vi "Kinematics_Wheel Deltas to Twist.vi"(9 "WheelDeltas":T2[](array[typedef]) {"Angle"."SIN" format="%13.4f"; "Angle"."COS" format="%13.4f"; "Angle"."VALUE" format="%13.4f"}, 11 "In SWERVE_DRIVE_KINEMATICS":T4 {"SavedModuleStates"."Angle"."SIN" format="%13.4f"; "SavedModuleStates"."Angle"."COS" format="%13.4f"; "SavedModuleStates"."Angle"."VALUE" format="%13.4f"; "PrevCoR"."Y" format="%14.3f"; "PrevCoR"."X" format="%14.3f"; "Modules"."Y" format="%14.3f"; "Modules"."X" format="%14.3f"}) -> (1 "Size Error Out":bool, 3 "Twist2d Out":T1)   [LabVIEW 2023, in "Swerve_Odometry_SEN.lvlib"]
doc: "Performs forward kinematics to return the resulting chassis state from the given module states. This method is often used for odometry -- determining the robot's position on the field using data from the real-world speed and angle of each module on the robot.\n\n\nParameters: \n - in Swerve Drive Kinematics - Swerve drive kinematics data structure\n - wheelDeltas - An array of the latest change in position of the modules (as a SwerveModulePosition type) as measured from respective encoders and gyros. The order of the swerve module states should be same as passed into the constructor of this class.\n\nReturns:\n - The resulting twist2d."
uses:
  Swerve_Odometry_SEN.lvlib
  Cluster_SWERVE_DRIVE_KINEMATICS.ctl
  <vilib>/Analysis/Matrix/Datatypes/RealMatrix.ctl
  Cluster_TRANSLATION2D.ctl
  Cluster_SWERVE_DRIVE_MODULE_STATE.ctl
  Cluster_ROTATION2D.ctl
  Cluster_SWERVE_DRIVE_MODULE_POSITION.ctl
  Cluster_TWIST2D.ctl
  <vilib>/Analysis/Matrix/Numeric/Multiply/Multiply - RM,RM.vi
  <vilib>/Analysis/Matrix/NI_Matrix.lvlib
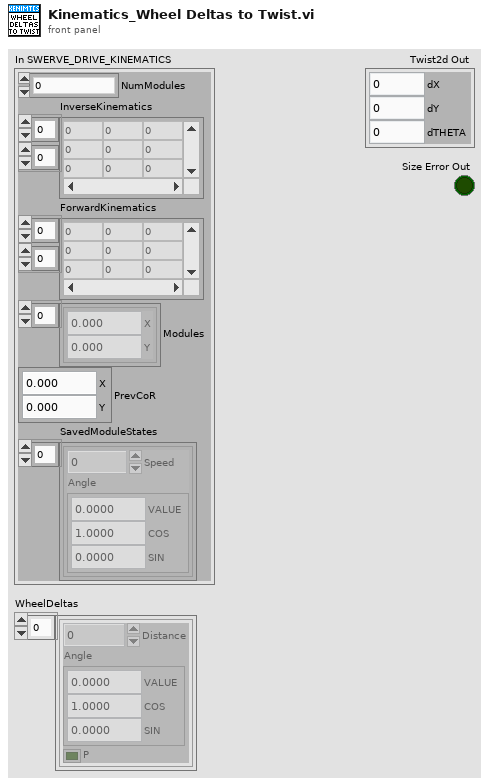
[diagram p1: front panel]
types:
  T1 = typedef "Swerve_Odometry_SEN.lvlib/Cluster_TWIST2D.ctl" = cluster{"dX":dbl, "dY":dbl, "dTHETA":dbl}
  T2 = typedef "Swerve_Odometry_SEN.lvlib/Cluster_SWERVE_DRIVE_MODULE_POSITION.ctl" = cluster{"Distance":dbl, "Angle":T3, "P":bool}
  T3 = typedef "Swerve_Odometry_SEN.lvlib/Cluster_ROTATION2D.ctl" = cluster{"VALUE":dbl, "COS":dbl, "SIN":dbl}
  T4 = typedef "Swerve_Odometry_SEN.lvlib/Cluster_SWERVE_DRIVE_KINEMATICS.ctl" = cluster{"NumModules":i32, "InverseKinematics":T5, "ForwardKinematics":T5, "Modules":T6[], "PrevCoR":T6, "SavedModuleStates":T7[]}
  T5 = typedef "NI_Matrix.lvlib/RealMatrix.ctl" = dbl[][]
  T6 = typedef "Swerve_Odometry_SEN.lvlib/Cluster_TRANSLATION2D.ctl" = cluster{"X":dbl, "Y":dbl}
  T7 = typedef "Swerve_Odometry_SEN.lvlib/Cluster_SWERVE_DRIVE_MODULE_STATE.ctl" = cluster{"Speed":dbl, "Angle":T3}
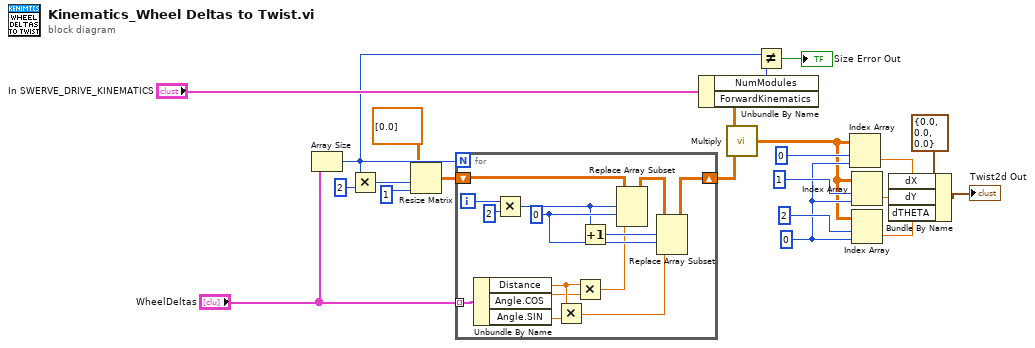
[diagram p0: block diagram]
diagram:
  w14 = 0 ("index (col)")
  n1 = Array Size(array="WheelDeltas") -> (size(s)=w11:i32)
  n2 = Multiply(x=w11, y=2) -> (x*y=w6:i32)
  n3 = Resize Matrix(1:1 ("number of columns"), 2:w6, 4:T5 [[0.0]] ("matrix")) -> (0:w8:T5)
  n4 = for {
    N: w11 -> [_]
    shift-right: [w28] -> w19
    shift-left: w8 -> [w36]
    tunnel: "WheelDeltas" -> [w30] mode=indexing
    i -> [w34]
    w35 = 0 ("disabled index (col)")
    n5 = Unbundle By Name(w30) -> ("Distance"=w27:dbl, "Angle.COS"=w26:dbl, "Angle.SIN"=w25:dbl)
    n6 = Multiply(x=w34, y=2) -> (x*y=w32:i32)
    n7 = Multiply(x=w27, y=w25) -> (x*y=w23:dbl)
    n8 = Multiply(x=w27, y=w26) -> (x*y=w24:dbl)
    n9 = Increment(x=w32) -> (x+1=w31:i32)
    n10 = Replace Array Subset(array=w36, new element=w24, index (row)=w32, index (col)=w35) -> (w29:T5)
    n11 = Replace Array Subset(array=w29, new element=w23, index (row)=w31, index (col)=w35) -> (w28:T5)
  }
  n12 = Unbundle By Name("In SWERVE_DRIVE_KINEMATICS") -> ("NumModules"=w12:i32, "ForwardKinematics"=w20:T5)
  n13 = call-poly <vilib>:"Multiply.vi"("Real Matrix B"=w19, "Real Matrix A"=w20) -> ("A * B"=w13:T5)
  n14 = Not Equal?(x=w11, y=w12) -> (x != y?=→"Size Error Out":bool)
  n15 = Index Array(array=w13, index (row)=0, index (col)=w14) -> (element=w4:dbl)
  n16 = Index Array(array=w13, index (row)=1, index (col)=w14) -> (element=w3:dbl)
  n17 = Index Array(array=w13, index (row)=2, index (col)=w14) -> (element=w2:dbl)
  n18 = Bundle By Name(cluster=T1 {"dX"=0.0, "dY"=0.0, "dTHETA"=0.0} ("Twist2d 2"), "dX"=w4, "dY"=w3, "dTHETA"=w2) -> (→"Twist2d Out":T1)
